vi "Perform Action.vi"(8 "error in (no error)":errorcluster, 10 "Input":variant, 11 "Sample PI Control in":refnum<class "Sample PI Control.lvclass">) -> (0 "error out":errorcluster, 2 "Output":variant, 3 "Sample PI Control out":refnum<class "Sample PI Control.lvclass">)   [LabVIEW 2023, in "Sample PI Control.lvclass"]
uses:
  Sample PI Control.lvclass
  D:/git/HAL/HAL GOOP4/Task Base/Task Base.lvclass
  Task Base/Task Base.lvclass/Task Base.ctl
  Sample PI Control.lvclass/Sample PI Control.ctl
  <vilib>/addons/control/pid/pid.llb/PID (DBL).vi
  Measure and Stimulus Subsystems/Measure and Stimulus Subsystems.lvclass
  Task Base/Task Base.lvclass
  <vilib>/addons/control/pid/NI_PID_pid.lvlib
  D:/git/HAL/HAL GOOP4/Sample Tasks/Sample PI Control/Sample PI Control.lvclass
panel:
  out "Powersensor Scalar":dbl
  out "Photosensor Waveform Chart":waveform(dbl)(graph)
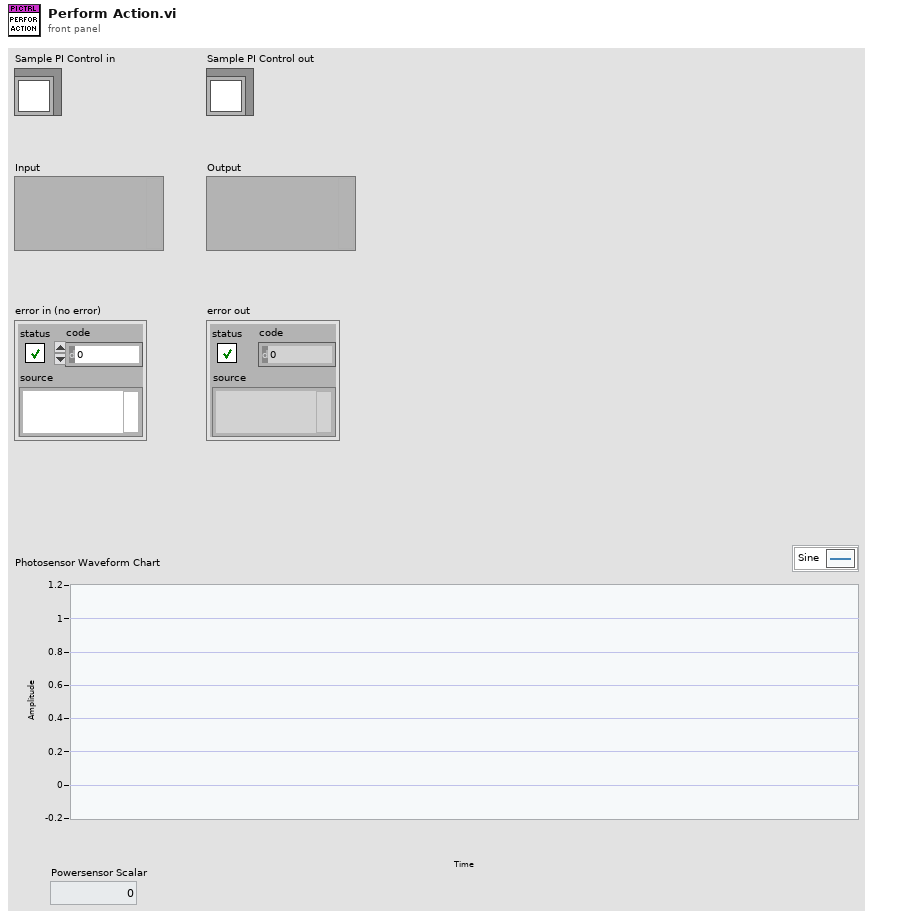
[diagram p1: front panel]
types:
  T1 = cluster{"Stop Notifier":refnum<notifier>, "Data Notifier":refnum<notifier>}
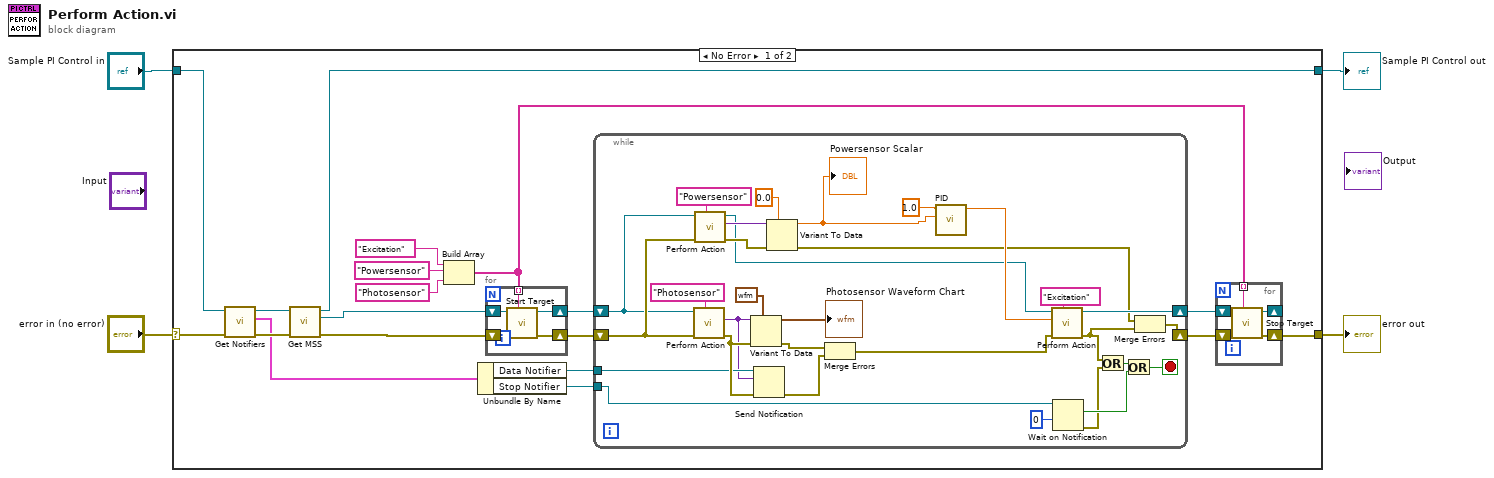
[diagram p0: block diagram]
diagram:
  n1 = case shown="No Error" "error in (no error)" {
    selector: "error in (no error)" -> [w20 w65]
    tunnel: [w16 w65] -> w3
    tunnel: [w15 w64] -> w1
    tunnel: "Sample PI Control in" -> [w8 w64]
    frame No Error {
      n2 = call "Get Notifiers.vi"("error in (no error)"=w20, "Task Base in"=w8) -> ("error out"=w14:errorcluster, "Notifier"=w9:T1, "Task Base out"=w13:refnum<class "Sample PI Control.lvclass">)  [unwired: 7 in]
      n3 = call "Get MSS.vi"("error in (no error)"=w14, "Task Base in"=w13) -> ("error out"=w19:errorcluster, "MSS"=w18:refnum<class "Measure and Stimulus Subsystems.lvclass">, "Task Base out"=w15:refnum<class "Sample PI Control.lvclass">)  [unwired: 7 in]
      n4 = Build Array("Excitation" ("Target Ident"), "Powersensor" ("Target Identifier"), "Photosensor" ("Target Identifier")) -> (w5:string[])
      n5 = Unbundle By Name(w9) -> ("Data Notifier"=w6:refnum<notifier>, "Stop Notifier"=w7:refnum<notifier>)
      n6 = for {
        shift-right: [w28] -> w23
        shift-left: w19 -> [w26]
        shift-right: [w27] -> w22
        shift-left: w18 -> [w25]
        tunnel: w5 -> [w24] mode=indexing
        n7 = call "Start Target.vi"("Target Ident"=w24, "Error In"=w26, "reference in"=w25) -> ("Error Out"=w28:errorcluster, "reference out"=w27:refnum<class "Measure and Stimulus Subsystems.lvclass">)  [unwired: 7 in]
      }
      n8 = while {
        shift-right: [w44] -> w21
        shift-left: w23 -> [w50]
        shift-right: [w52] -> w17
        shift-left: w22 -> [w49]
        tunnel: w7 -> [w33]
        tunnel: w6 -> [w37]
        stop <- w42 stop-if-true
        n9 = call "Perform Action.vi"("Target Ident"="Photosensor" ("Target Identifier"), "Error In"=w50, "reference in"=w49) -> ("Error Out"=w39:errorcluster, "Output"=w36:variant)  [unwired: 6 in, 1 out]
        n10 = call "Perform Action.vi"("Target Ident"="Powersensor" ("Target Identifier"), "Error In"=w50, "reference in"=w49) -> ("Error Out"=w56:errorcluster, "Output"=w54:variant, "reference out"=w45:refnum<class "Measure and Stimulus Subsystems.lvclass">)  [unwired: 6 in]
        n11 = Variant To Data(error in=w39, type=waveform(dbl) {"t0"=timestamp(0 s since 1904-01-01), "dt"=1.0, "Y"=[]} ("Waveform"), Variant=w36) -> (data=→"Photosensor Waveform Chart":waveform(dbl), error out=w35:errorcluster)
        n12 = Send Notification(notification=w36, notifier=w37, error in (no error)=w39) -> (error out=w34:errorcluster)  [unwired: 1 out]
        n13 = Variant To Data(error in=w56, type=0.0, Variant=w54) -> (data=w47:dbl, error out=w43:errorcluster)
        "Powersensor Scalar" <- w47
        n14 = Merge Errors(w35, w34) -> (w29:errorcluster)
        n15 = call-poly <vilib>:"PID.vi"("process variable"=w47, "setpoint"=1.0) -> ("output"=w46:dbl)  [unwired: 8 in, 1 out]
        n16 = call "Perform Action.vi"("Target Ident"="Excitation", "Error In"=w29, "Input"=w46, "reference in"=w45) -> ("Error Out"=w30:errorcluster, "reference out"=w52:refnum<class "Measure and Stimulus Subsystems.lvclass">)  [unwired: 5 in, 1 out]
        n17 = Wait on Notification(notifier=w33, timeout in ms (-1)=0) -> (notification=w38:bool, error out=w32:errorcluster)  [unwired: 2 in, 2 out]
        n18 = Or(x=w30, y=w32) -> (x .or. y?=w31:bool)
        n19 = Or(x=w31, y=w38) -> (x .or. y?=w42:bool)
        n20 = Merge Errors(w43, w30) -> (w44:errorcluster)
      }
      n21 = for {
        shift-right: [w61] -> w16
        shift-left: w21 -> [w63]
        tunnel: w5 -> [w60] mode=indexing
        shift-right: [w59] -> _
        shift-left: w17 -> [w62]
        n22 = call "Stop Target.vi"("Target Ident"=w60, "Error In"=w63, "reference in"=w62) -> ("Error Out"=w61:errorcluster, "reference out"=w59:refnum<class "Measure and Stimulus Subsystems.lvclass">)  [unwired: 7 in]
      }
    }
    frame Error {
    }
  }
  "error out" <- w3
  "Sample PI Control out" <- w1
